vi "Generate_WayPoints_Hopping_DoubleLSV.vi"(11 "Input Cluster":T2={"Scan Rate (um/s)"=15.0, "X Start"=15.0, "X End"=15.0, "Y Start"=15.0, "Y End"=15.0, " Z Start"=15.0, "HoppingDistance"=1.0, "V"=15.0, "Z End"=15.0, "Approach Rate Hopping (um/s)"=15.0, "Retrack Rate (um/s)"=15.0, "V 2"=15.0, "Approach Rate (um/s)"=15.0, "CV Rate / V/s"=15.0, "V 1"=15.0, "HoldTime1/s"=15.0}) -> (0 "output cluster":T1)   [LabVIEW 2023]
uses:
  TypeDefs/WayPointCluster.ctl
  User_Vi/Settings.vi
panel:
  in  "WayPointCluster":T1
  out "Y  P":dbl
  out "X  P":dbl
  out "HoppingDistanceX":dbl
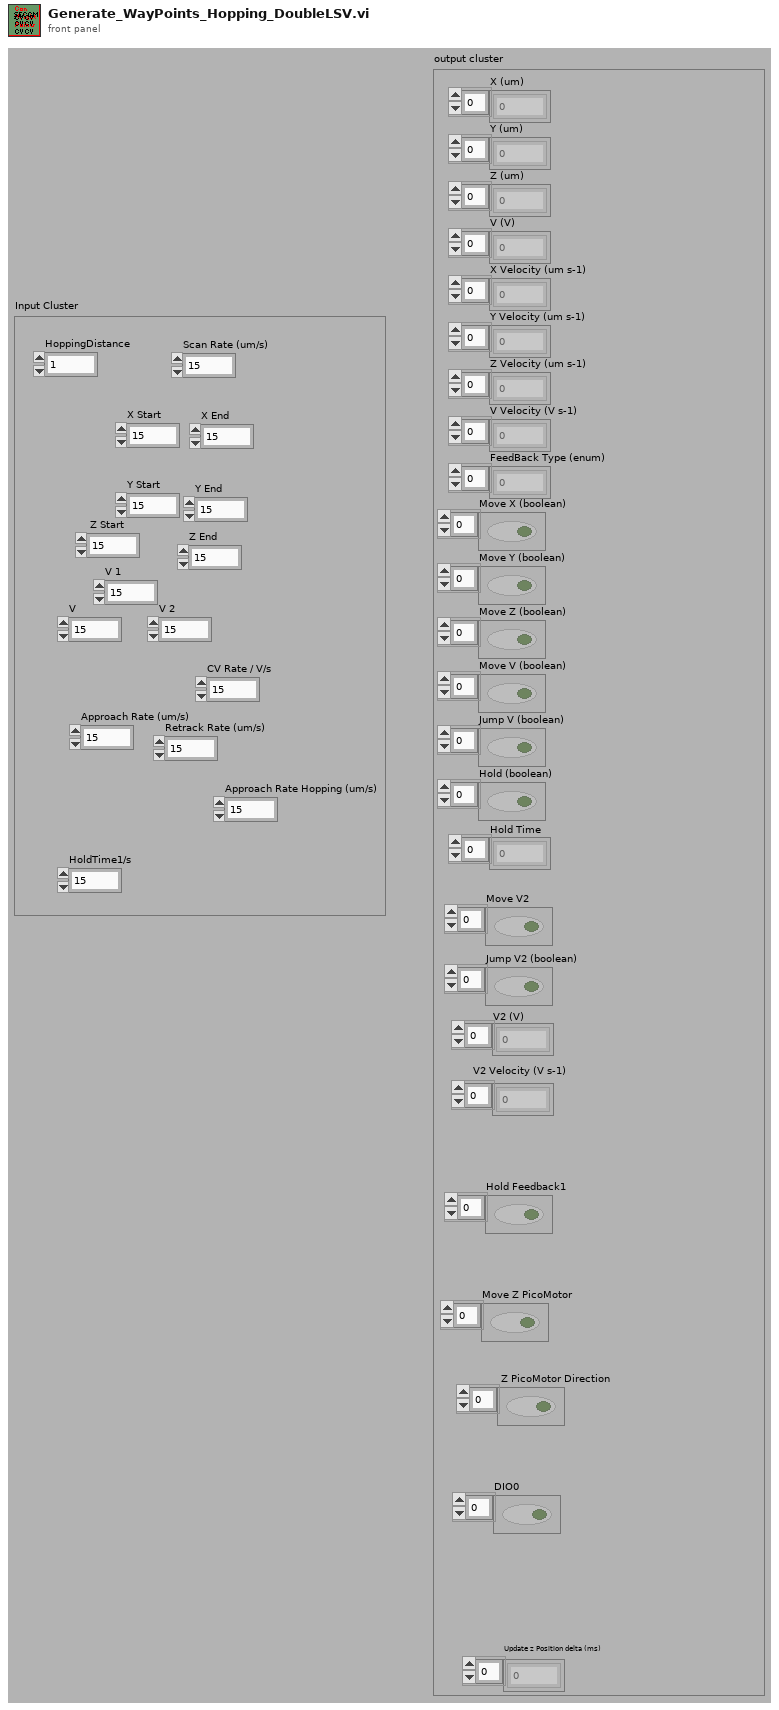
[diagram p1: front panel]
types:
  T1 = typedef "WayPointCluster.ctl" = cluster{"X (um)":dbl[], "Y (um)":dbl[], "Z (um)":dbl[], "V (V)":dbl[], "X Velocity (um s-1)":dbl[], "Y Velocity (um s-1)":dbl[], "Z Velocity (um s-1)":dbl[], "V Velocity (V s-1)":dbl[], "FeedBack Type (enum)":u16[], "Move X (boolean)":bool[], "Move Y (boolean)":bool[], "Move Z (boolean)":bool[], "Move V (boolean)":bool[], "Jump V (boolean)":bool[], "Hold (boolean)":bool[], "Hold Time":u32[], "V2 (V)":dbl[], "Move V2":bool[], "V2 Velocity (V s-1)":dbl[], "Jump V2 (boolean)":bool[], "Update z Position delta (ms)":i16[], "Hold Feedback1":bool[], "Move Z PicoMotor":bool[], " Z PicoMotor Direction":bool[], "DIO0":bool[]}
  T2 = cluster{"Scan Rate (um/s)":dbl, "X Start":dbl, "X End":dbl, "Y Start":dbl, "Y End":dbl, " Z Start":dbl, "HoppingDistance":dbl, "V":dbl, "Z End":dbl, "Approach Rate Hopping (um/s)":dbl, "Retrack Rate (um/s)":dbl, "V 2":dbl, "Approach Rate (um/s)":dbl, "CV Rate / V/s":dbl, "V 1":dbl, "HoldTime1/s":dbl}
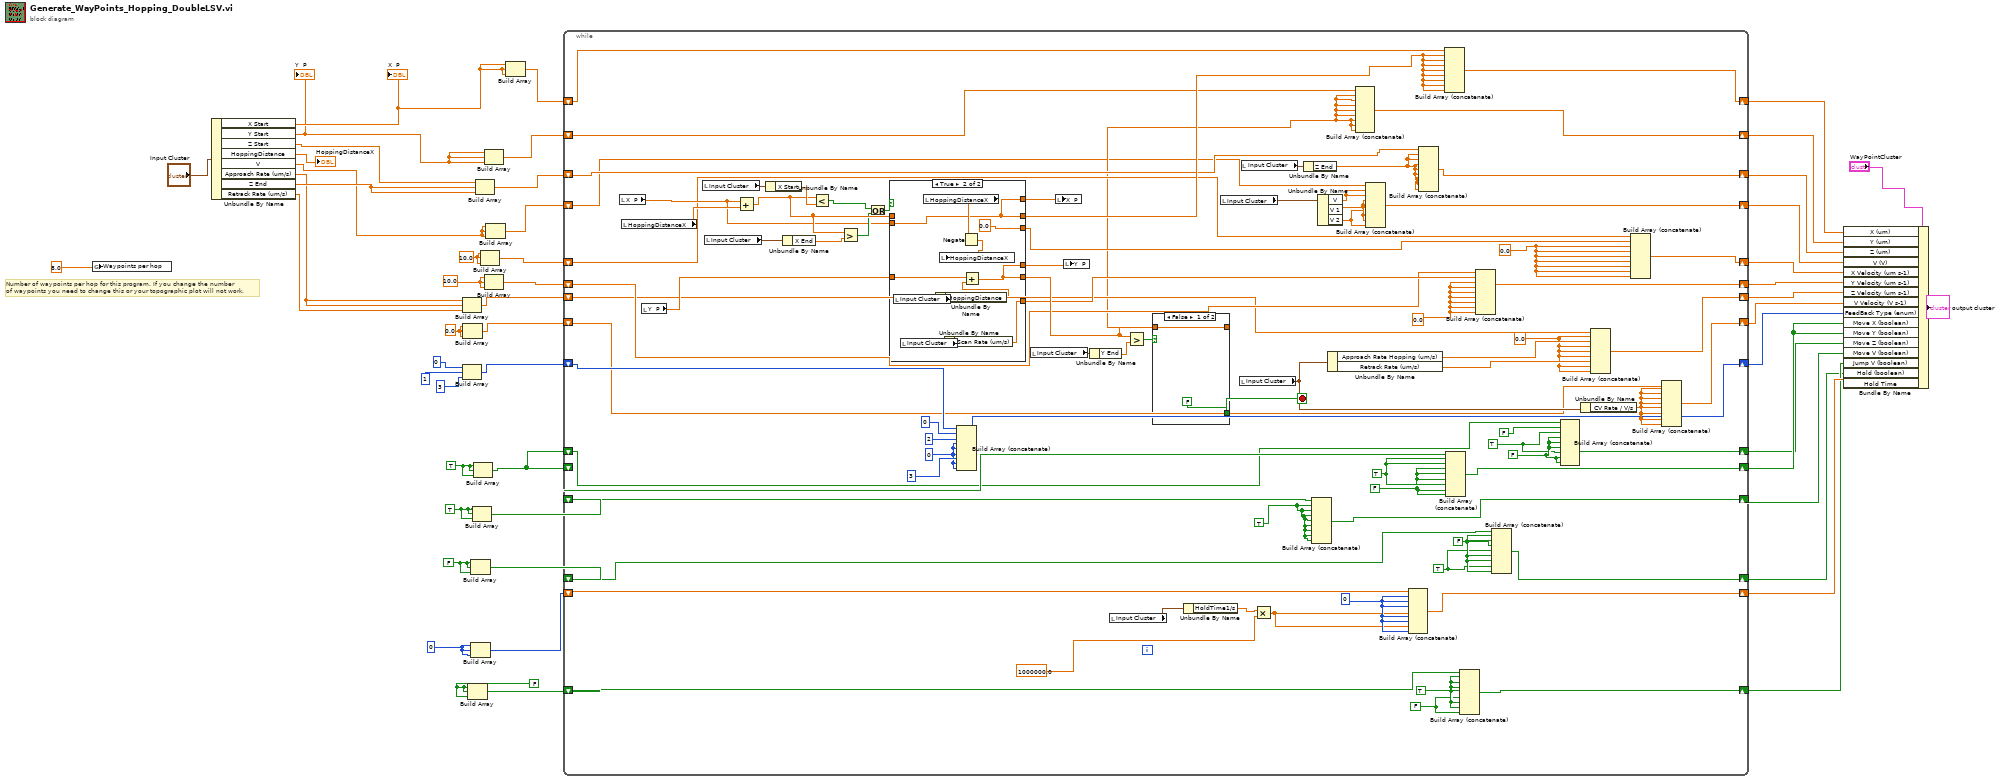
[diagram p0: block diagram]
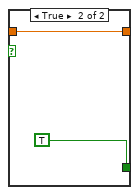
[diagram p2: hidden frame]
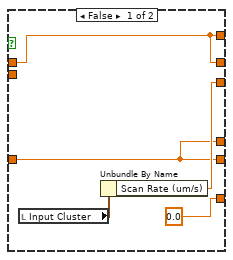
[diagram p3: hidden frame]
diagram:
  w15 = FALSE
  w18 = FALSE
  w17 = u32 0 ("element")
  w16 = TRUE
  w13 = TRUE
  w9 = 10.0 ("element")
  w10 = 10.0 ("element")
  w12 = 0.0 ("element")
  # "Number of waypoints per hop for this program. If you change the number\nof waypoints you need to change this or your topographic plot will not work."
  n1 = global write "Settings.vi" "Waypoints per hop"(8.0) -> ()
  n2 = Unbundle By Name("Input Cluster") -> ("X Start"=w31:dbl, "Y Start"=w30:dbl, "Z Start"=w32:dbl, "HoppingDistance"=→"HoppingDistanceX":dbl, "V"=w28:dbl, "Approach Rate (um/s)"=w11:dbl, "Z End"=w29:dbl, "Retrack Rate (um/s)"=w27:dbl)
  "X  P" <- w31
  "Y  P" <- w30
  n3 = Build Array(w11, w11, w27) -> (w39:dbl[])
  n4 = Build Array(u16 0 ("element"), u16 1 ("element"), u16 3 ("element")) -> (w35:u16[])
  n5 = Build Array(w12, w12, w12) -> (w37:dbl[])
  n6 = Build Array(w18, w18, w18) -> (w22:bool[])
  n7 = Build Array(w15, w15, w15) -> (w14:bool[])
  n8 = Build Array(w17, w17, w17) -> (w25:u32[])
  n9 = Build Array(w16, w16, w16) -> (w20:bool[])
  n10 = Build Array(w13, w13, w13) -> (w3:bool[])
  n11 = Build Array(w32, w29, w29) -> (w46:dbl[])
  n12 = Build Array(w9, w9, w9) -> (w42:dbl[])
  n13 = Build Array(w30, w30, w30) -> (w48:dbl[])
  n14 = Build Array(w10, w10, w10) -> (w41:dbl[])
  n15 = Build Array(w28, w28, w28) -> (w44:dbl[])
  n16 = Build Array(w31, w31, w31) -> (w50:dbl[])
  n17 = while {
    shift-right: [w112] -> w49
    shift-left: w50 -> [w61]
    shift-right: [w109] -> w47
    shift-left: w48 -> [w110]
    shift-right: [w107] -> w45
    shift-left: w46 -> [w108]
    shift-right: [w99] -> w43
    shift-left: w44 -> [w60]
    shift-right: [w98] -> w4
    shift-left: w42 -> [w105]
    shift-right: [w67] -> w40
    shift-left: w41 -> [w101]
    shift-right: [w96] -> w38
    shift-left: w39 -> [w97]
    shift-right: [w93] -> w36
    shift-left: w37 -> [w94]
    shift-right: [w132] -> w34
    shift-left: w35 -> [w133]
    shift-right: [w90] -> w24
    shift-left: w3 -> [w91]
    shift-right: [w85] -> w6
    shift-left: w14 -> [w86]
    shift-right: [w83] -> w23
    shift-left: w25 -> [w84]
    shift-right: [w79] -> w21
    shift-left: w22 -> [w80]
    shift-right: [w88] -> w5
    shift-left: w20 -> [w89]
    shift-right: [w57] -> w2
    shift-left: w3 -> [w58]
    stop <- w120 stop-if-true
    w55 = FALSE
    w54 = TRUE
    w78 = TRUE
    w103 = 0.0 ("element")
    w87 = TRUE
    w77 = FALSE
    w76 = u32 0 ("element")
    w73 = TRUE
    w74 = FALSE
    w71 = FALSE
    w72 = TRUE
    w53 = u16 0 ("element")
    w100 = 0.0 ("element")
    w66 = 0.0 ("element")
    n18 = local read "X  P"() -> (w119:dbl)
    n19 = local read "HoppingDistanceX"() -> (w134:dbl)
    n20 = local read "Y  P"() -> (w118:dbl)
    n21 = local read "Input Cluster"() -> (w136:T2)
    n22 = local read "Input Cluster"() -> (w135:T2)
    n23 = Add(x=w119, y=w134) -> (x+y=w126:dbl)
    n24 = Unbundle By Name(w136) -> ("X Start"=w129:dbl)
    n25 = Unbundle By Name(w135) -> ("X End"=w127:dbl)
    n26 = Less?(x=w126, y=w129) -> (x < y?=w128:bool)
    n27 = Greater?(x=w126, y=w127) -> (0:w125:bool)
    n28 = Or(x=w128, y=w125) -> (x .or. y?=w124:bool)
    n29 = case shown="True" w124 {
      tunnel: w126 -> [w141 _]
      tunnel: [w141 w147] -> w111
      tunnel: w119 -> [_ w147]
      tunnel: w118 -> [w142 w148]
      tunnel: [w142 w146] -> w117
      tunnel: [w144 0.0] -> w104
      tunnel: [0.0 w149] -> w102
      tunnel: [w142 w146] -> w116
      tunnel: [w141 w147] -> w115
      frame False {
        n30 = local read "Input Cluster"() -> (w145:T2)
        n31 = Unbundle By Name(w145) -> ("Scan Rate (um/s)"=w144:dbl)
      }
      frame True {
        n32 = local read "Input Cluster"() -> (w153:T2)
        n33 = local read "Input Cluster"() -> (w151:T2)
        n34 = local read "HoppingDistanceX"() -> (w155:dbl)
        n35 = Unbundle By Name(w153) -> ("HoppingDistance"=w152:dbl)
        n36 = Unbundle By Name(w151) -> ("Scan Rate (um/s)"=w149:dbl)
        n37 = Negate(x=w155) -> (-x=w154:dbl)
        n38 = local write "HoppingDistanceX"(w154) -> ()
        n39 = Add(x=w148, y=w152) -> (x+y=w146:dbl)
      }
    }
    n40 = Build Array (concatenate)(w133, u16 0 ("element"), u16 2 ("element"), w53, w53, w53, u16 3 ("element"), w53, w53) -> (w132:u16[])
    n41 = local read "Input Cluster"() -> (w123:T2)
    n42 = local write "X  P"(w115) -> ()
    n43 = local write "Y  P"(w116) -> ()
    n44 = Unbundle By Name(w123) -> ("Y End"=w122:dbl)
    n45 = local read "Input Cluster"() -> (w82:T2)
    n46 = Greater?(x=w117, y=w122) -> (0:w121:bool)
    n47 = case shown="False" w121 {
      tunnel: w117 -> [w138 w140]
      tunnel: [w138 w140] -> w62
      tunnel: [FALSE TRUE] -> w120
      frame False {
      }
      frame True {
      }
    }
    n48 = Unbundle By Name(w82) -> ("HoldTime1/s"=w81:dbl)
    n49 = local read "Input Cluster"() -> (w130:T2)
    n50 = local read "Input Cluster"() -> (w113:T2)
    n51 = local read "Input Cluster"() -> (w131:T2)
    n52 = Multiply(x=w81, y=1000000.0 ("element")) -> (x*y=w75:dbl)
    n53 = Unbundle By Name(w131) -> ("Z End"=w106:dbl)
    n54 = Build Array (concatenate)(w89, w87, w87, w87, w87, w87, w87, w87, w87) -> (w88:bool[])
    n55 = Unbundle By Name(w130) -> ("V"=w65:dbl, "V 1"=w64:dbl, "V 2"=w63:dbl)
    n56 = Unbundle By Name(w113) -> ("Approach Rate Hopping (um/s)"=w95:dbl, "Retrack Rate (um/s)"=w68:dbl)
    n57 = Build Array (concatenate)(w110, w62, w62, w62, w62, w62, w62, w62, w62) -> (w109:dbl[])
    n58 = Build Array (concatenate)(w60, w65, w65, w64, w64, w63, w64, w64, w63) -> (w99:dbl[])
    n59 = Build Array (concatenate)(w84, w76, w76, w76, w75, w76, w76, w75, w76) -> (w83:dbl[])
    n60 = Build Array (concatenate)(w108, w106, w106, w106, w106, w106, w106, w106, w106) -> (w107:dbl[])
    n61 = Build Array (concatenate)(w61, w111, w111, w111, w111, w111, w111, w111, w111) -> (w112:dbl[])
    n62 = Build Array (concatenate)(w91, w72, w72, w71, w71, w71, w72, w71, w71) -> (w90:bool[])
    n63 = Build Array (concatenate)(w80, w78, w78, w78, w78, w77, w78, w78, w77) -> (w79:bool[])
    n64 = Build Array (concatenate)(w101, w102, w100, w100, w100, w100, w100, w100, w100) -> (w67:dbl[])
    n65 = Build Array (concatenate)(w86, w74, w74, w74, w73, w74, w74, w73, w74) -> (w85:bool[])
    n66 = Build Array (concatenate)(w58, FALSE, w54, w55, w55, w55, w54, w55, w55) -> (w57:bool[])
    n67 = Unbundle By Name(w113) -> ("CV Rate / V/s"=w92:dbl)
    n68 = Build Array (concatenate)(w97, w66, w95, w66, w66, w66, w68, w66, w66) -> (w96:dbl[])
    n69 = Build Array (concatenate)(w105, w104, w103, w103, w103, w103, w103, w103, w103) -> (w98:dbl[])
    n70 = Build Array (concatenate)(w94, w92, w92, w92, w92, w92, w92, w92, w92) -> (w93:dbl[])
  }
  n71 = Bundle By Name(cluster="WayPointCluster", "X (um)"=w49, "Y (um)"=w47, "Z (um)"=w45, "V (V)"=w43, "X Velocity (um s-1)"=w4, "Y Velocity (um s-1)"=w40, "Z Velocity (um s-1)"=w38, "V Velocity (V s-1)"=w36, "FeedBack Type (enum)"=w34, "Move X (boolean)"=w24, "Move Y (boolean)"=w24, "Move Z (boolean)"=w2, "Move V (boolean)"=w5, "Jump V (boolean)"=w21, "Hold (boolean)"=w6, "Hold Time"=w23) -> (→"output cluster":T1)
